vi "lia_fpgaNOFIFO.vi"() -> ()   [LabVIEW 2009]
uses:
  <vilib>/eio/EIONode/EIONode.xnode
  <vilib>/rvi/eio/nirviEIOImplementation/nirviEIOImplementation.xnode
  <vilib>/rvi/eio/common/nirviEmuTemplateMethod_noerrors.vi
  <vilib>/rvi/eio/common/nirviEmuClasses.ctl
panel:
  out "X_fpga 3":i32
  out "Y_fpga 3":i32
  in  "beta 3":i32
  in  "Phase Shift Cos 3":u32
  out "Accumulator Value 3":u32
  in  "Signal Amplitude 3":u16
  in  "Phase Shift 3":u32
  in  "Accumulator Increment 3":u32
  out "X_fpga 2":i32
  out "Y_fpga 2":i32
  in  "beta 2":i32
  in  "Phase Shift Cos 2":u32
  out "Accumulator Value 2":u32
  in  "Signal Amplitude 2":u16
  in  "Phase Shift 2":u32
  in  "Accumulator Increment 2":u32
  out "X_fpga 1":i32
  out "Y_fpga 1":i32
  in  "beta 1":i32
  in  "Phase Shift Cos 1":u32
  in  "stop":bool
  out "Actual Gen Rate (ticks)":u32
  in  "Update Rate (ticks)":u32
  out "Accumulator Value 1":u32
  in  "Signal Amplitude 1":u16
  in  "Phase Shift 1":u32
  in  "Accumulator Increment 1":u32
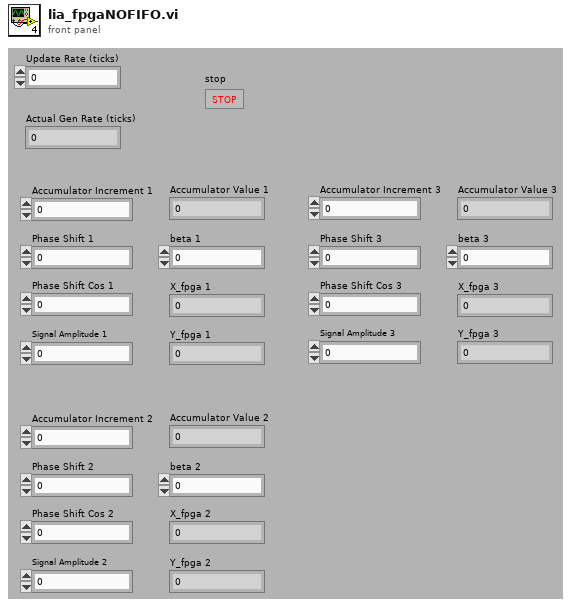
[diagram p1: front panel]
types:
  T1 = typedef "nirviEmuClasses.ctl" = enum16{"IO Read", "IO Write", "Method", "Property Read", "Property Write"}
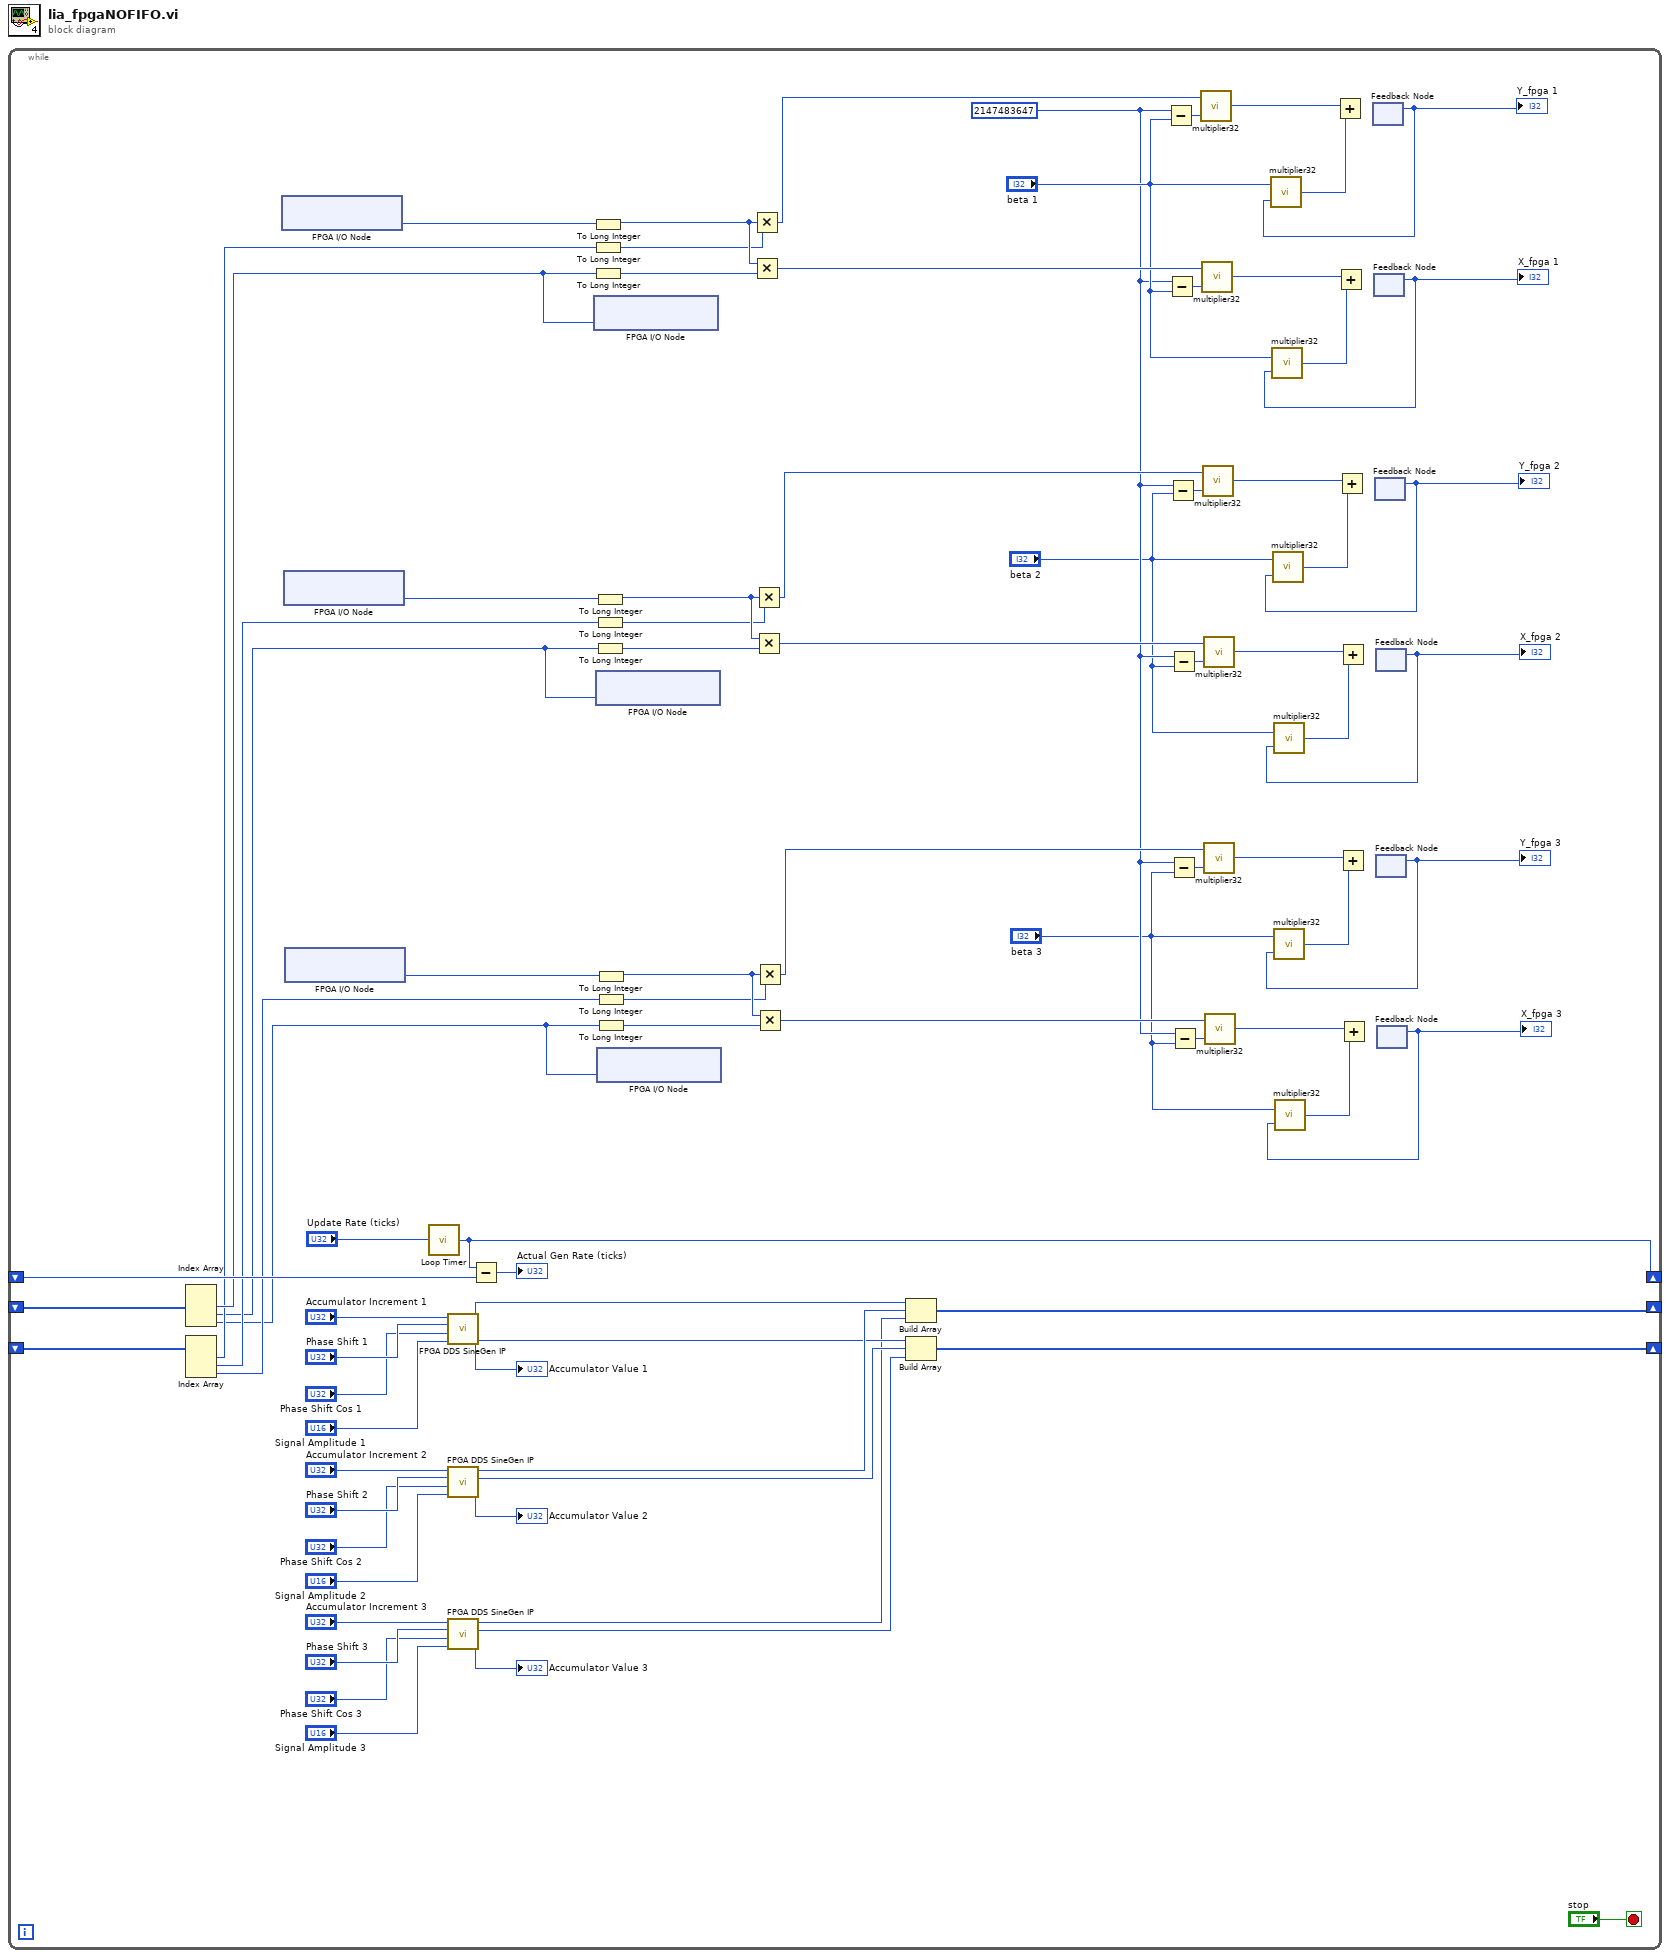
[diagram p0: block diagram]
diagram:
  n1 = while {
    shift-right: [w57] -> _
    shift-left: _ -> [w55]
    shift-right: [w85] -> _
    shift-left: _ -> [w83]
    shift-right: [w56] -> _
    shift-left: _ -> [w53]
    stop <- "stop" stop-if-true
    w3 = 2147483647
    n2 = Index Array(array=w55) -> (element #1=w54:i16, element #2=w38:i16, element #3=w5:i16)  [unwired: 3 in]
    n3 = Index Array(array=w53) -> (element #1=w52:i16, element #2=w39:i16, element #3=w6:i16)  [unwired: 3 in]
    n4 = xnode "FPGA I/O Node"() -> ("Connector0/AI0"=w70:i16)  [unwired: 1 in, 1 out]
    n5 = xnode "FPGA I/O Node"() -> ("Connector0/AI1"=w43:i16)  [unwired: 1 in, 1 out]
    n6 = xnode "FPGA I/O Node"() -> ("Connector0/AI2"=w14:i16)  [unwired: 1 in, 1 out]
    n7 = call "Loop Timer"("Count(Ticks)"="Update Rate (ticks)") -> ("Tick Count(Ticks)"=w85:u32)
    n8 = call "FPGA DDS SineGen IP.vi"("Signal Amplitude (x 2^15)"="Signal Amplitude 1", 9:"Phase Shift Cos 1", "Phase Shift"="Phase Shift 1", "Accumulator Increment"="Accumulator Increment 1") -> ("Accumulator Value"=→"Accumulator Value 1":u32, "Cos output"=w59:i16, "Sin output"=w61:i16)  [unwired: 5 in]
    n9 = call "FPGA DDS SineGen IP.vi"("Signal Amplitude (x 2^15)"="Signal Amplitude 2", 9:"Phase Shift Cos 2", "Phase Shift"="Phase Shift 2", "Accumulator Increment"="Accumulator Increment 2") -> ("Accumulator Value"=→"Accumulator Value 2":u32, "Cos output"=w58:i16, "Sin output"=w60:i16)  [unwired: 5 in]
    n10 = call "FPGA DDS SineGen IP.vi"("Signal Amplitude (x 2^15)"="Signal Amplitude 3", 9:"Phase Shift Cos 3", "Phase Shift"="Phase Shift 3", "Accumulator Increment"="Accumulator Increment 3") -> ("Accumulator Value"=→"Accumulator Value 3":u32, "Cos output"=w23:i16, "Sin output"=w24:i16)  [unwired: 5 in]
    n11 = Subtract(x=w85, y=w83) -> (x-y=→"Actual Gen Rate (ticks)":u32)
    n12 = To Long Integer(number=w70) -> (32bit integer=w69:i32)
    n13 = To Long Integer(number=w52) -> (32bit integer=w68:i32)
    n14 = To Long Integer(number=w54) -> (32bit integer=w67:i32)
    n15 = xnode "FPGA I/O Node"("Connector0/AO0"=w54) -> ()  [unwired: 1 in, 1 out]
    n16 = To Long Integer(number=w43) -> (32bit integer=w42:i32)
    n17 = To Long Integer(number=w39) -> (32bit integer=w41:i32)
    n18 = To Long Integer(number=w38) -> (32bit integer=w40:i32)
    n19 = xnode "FPGA I/O Node"("Connector0/AO1"=w38) -> ()  [unwired: 1 in, 1 out]
    n20 = To Long Integer(number=w14) -> (32bit integer=w13:i32)
    n21 = To Long Integer(number=w6) -> (32bit integer=w12:i32)
    n22 = To Long Integer(number=w5) -> (32bit integer=w11:i32)
    n23 = xnode "FPGA I/O Node"("Connector0/AO2"=w5) -> ()  [unwired: 1 in, 1 out]
    n24 = Multiply(x=w69, y=w68) -> (x*y=w37:i32)
    n25 = Multiply(x=w69, y=w67) -> (x*y=w36:i32)
    n26 = Multiply(x=w42, y=w41) -> (x*y=w35:i32)
    n27 = Multiply(x=w42, y=w40) -> (x*y=w34:i32)
    n28 = Multiply(x=w13, y=w12) -> (x*y=w10:i32)
    n29 = Multiply(x=w13, y=w11) -> (x*y=w9:i32)
    n30 = Build Array(w61, w60, w24) -> (w57:i16[])
    n31 = Build Array(w59, w58, w23) -> (w56:i16[])
    n32 = Subtract(x=w3, y="beta 1") -> (x-y=w76:i32)
    n33 = Subtract(x=w3, y="beta 1") -> (x-y=w72:i32)
    n34 = Subtract(x=w3, y="beta 2") -> (x-y=w49:i32)
    n35 = Subtract(x=w3, y="beta 2") -> (x-y=w45:i32)
    n36 = Subtract(x=w3, y="beta 3") -> (x-y=w20:i32)
    n37 = Subtract(x=w3, y="beta 3") -> (x-y=w16:i32)
    n38 = call "multiplier32.vi"("Y"=w76, "X"=w37) -> ("XY"=w77:i32)
    n39 = call "multiplier32.vi"("Y"=w72, "X"=w36) -> ("XY"=w73:i32)
    n40 = call "multiplier32.vi"("Y"=w49, "X"=w35) -> ("XY"=w50:i32)
    n41 = call "multiplier32.vi"("Y"=w45, "X"=w34) -> ("XY"=w46:i32)
    n42 = call "multiplier32.vi"("Y"=w20, "X"=w10) -> ("XY"=w21:i32)
    n43 = call "multiplier32.vi"("Y"=w16, "X"=w9) -> ("XY"=w17:i32)
    n44 = feedback #1() -> (w33:i32)  [unwired: 1 in]
    "Y_fpga 1" <- w33
    n45 = call "multiplier32.vi"("Y"=w33, "X"="beta 1") -> ("XY"=w75:i32)
    n46 = Add(x=w77, y=w75) -> (x+y=w78:i32)
    n47 = feedback #2() -> (w32:i32)  [unwired: 1 in]
    "X_fpga 1" <- w32
    n48 = call "multiplier32.vi"("Y"=w32, "X"="beta 1") -> ("XY"=w71:i32)
    n49 = Add(x=w73, y=w71) -> (x+y=w74:i32)
    n50 = feedback #3() -> (w31:i32)  [unwired: 1 in]
    "Y_fpga 2" <- w31
    n51 = call "multiplier32.vi"("Y"=w31, "X"="beta 2") -> ("XY"=w48:i32)
    n52 = Add(x=w50, y=w48) -> (x+y=w51:i32)
    n53 = feedback #4() -> (w30:i32)  [unwired: 1 in]
    "X_fpga 2" <- w30
    n54 = call "multiplier32.vi"("Y"=w30, "X"="beta 2") -> ("XY"=w44:i32)
    n55 = Add(x=w46, y=w44) -> (x+y=w47:i32)
    n56 = feedback #5() -> (w8:i32)  [unwired: 1 in]
    "Y_fpga 3" <- w8
    n57 = call "multiplier32.vi"("Y"=w8, "X"="beta 3") -> ("XY"=w19:i32)
    n58 = Add(x=w21, y=w19) -> (x+y=w22:i32)
    n59 = feedback #6() -> (w7:i32)  [unwired: 1 in]
    "X_fpga 3" <- w7
    n60 = call "multiplier32.vi"("Y"=w7, "X"="beta 3") -> ("XY"=w15:i32)
    n61 = Add(x=w17, y=w15) -> (x+y=w18:i32)
  }
